vi "1-x-dist.vi"(0 "p_LN":T1, 5 "x":dbl, 11 "error in":errorcluster caption="err in") -> (4 "p_LN":T1, 6 "x":dbl, 8 "f(x)":dbl, 10 "F(x)":dbl=0.5 format="%.6g", 15 "error out":errorcluster caption="err out")   [LabVIEW 2010, in "lv_02.lvlib"]
uses:
  p_5E1_LN.ctl
  <vilib>/gmath/statdist.llb/Normal CDF.vi
  <vilib>/gmath/statdist.llb/Normal PDF.vi
  lv_02.lvlib
  <vilib>/gmath/NI_Gmath.lvlib
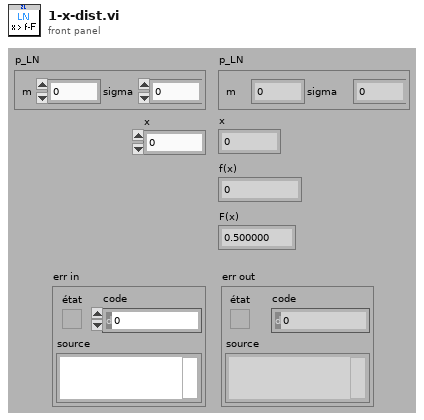
[diagram p1: front panel]
types:
  T1 = typedef "lv_02.lvlib/p_5E1_LN.ctl" = cluster{"m":dbl, "sigma":dbl}
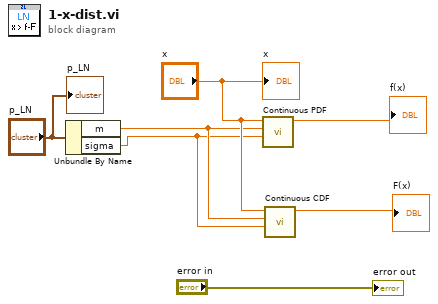
[diagram p0: block diagram]
diagram:
  n1 = Unbundle By Name("p_LN") -> ("m"=w4:dbl, "sigma"=w3:dbl)
  n2 = call-poly <vilib>:"Continuous PDF.vi"("std"=w3, "mean"=w4, "x"="x") -> ("pdf(x)"=→"f(x)":dbl)  [unwired: 7 in, 1 out]
  n3 = call-poly <vilib>:"Continuous CDF.vi"("std"=w3, "mean"=w4, "x"="x") -> ("cdf(x)"=→"F(x)":dbl)  [unwired: 7 in, 1 out]
  "error out" <- "error in"
  "p_LN" <- "p_LN"
  "x" <- "x"
